vi "Verifica_Correcao_CUP.vi"(3 "Erro max":i16, 4 "Pos Atual":i16, 5 "Azimute":u16) -> (1 "Corrigir?":bool)   [LabVIEW 2018]
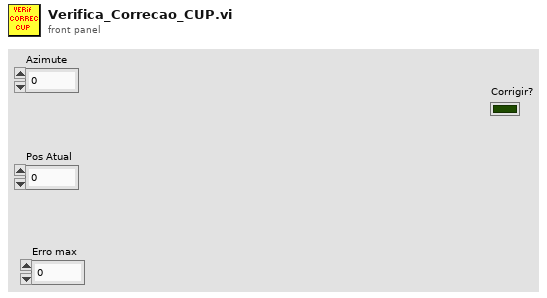
[diagram p1: front panel]
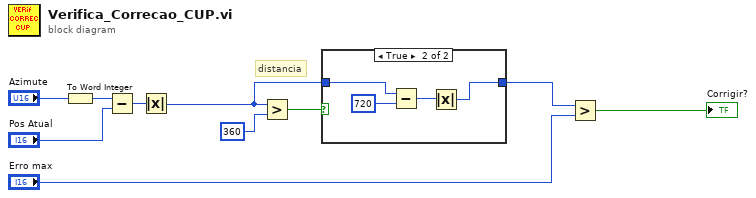
[diagram p0: block diagram]
diagram:
  # "distancia"
  n1 = To Word Integer(number="Azimute") -> (16bit integer=w1:i16)
  n2 = Subtract(x=w1, y="Pos Atual") -> (x-y=w9:i16)
  n3 = Absolute Value(x=w9) -> (abs(x)=w6:i16)
  n4 = Greater?(x=w6, y=i16 360) -> (0:w7:bool)
  n5 = case shown="True" w7 {
    tunnel: w6 -> [w11 w15]
    tunnel: [w11 w12] -> w5
    frame False {
    }
    frame True {
      n6 = Subtract(x=w15, y=i16 720) -> (x-y=w13:i16)
      n7 = Absolute Value(x=w13) -> (abs(x)=w12:i16)
    }
  }
  n8 = Greater?(x=w5, y="Erro max") -> (0:→"Corrigir?":bool)
